vi "Go Home.vi"() -> ()   [LabVIEW 2017]
uses:
  Go Home State type def.ctl
panel:
  out "X-axis distance":dbl
  out "Y-axis distance":dbl
  in  "stop":bool
  out "Motor Status":cluster{"Homing Freq":dbl, "Homing Duty %":dbl} {"Homing Duty %" format="%#_13g"; "Homing Freq" format="%#_13g"}
  in  "Homing Duty %":dbl format="%#_13g"
  in  "Homing Freq":dbl format="%#_13g"
  in  "error in (no error)":errorcluster
  out "error out":errorcluster
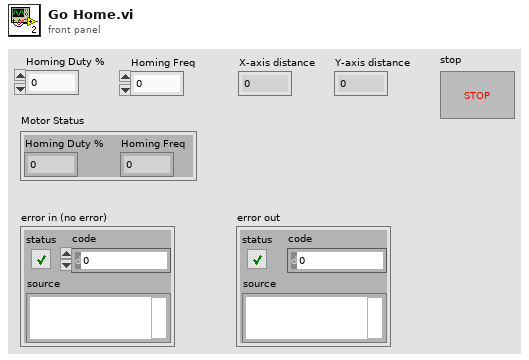
[diagram p1: front panel]
types:
  T1 = typedef "Go Home State type def.ctl" = enum16{"Stop Motor", "Read Input", "Drive Y", "Drive X"}
  T2 = typedef "Encoder Count Direction Enum.ctl" = enum16{"Counting Up", "Counting Down"}
  T3 = cluster{"Y-axis rev count":dbl, "Y-axis distance":dbl, "X-axis rev count":dbl, "X-axis distance":dbl, "Y-axis direction":T2, "X-axis direction":T2, "X-counter val":i32, "Y-counter val":i32}
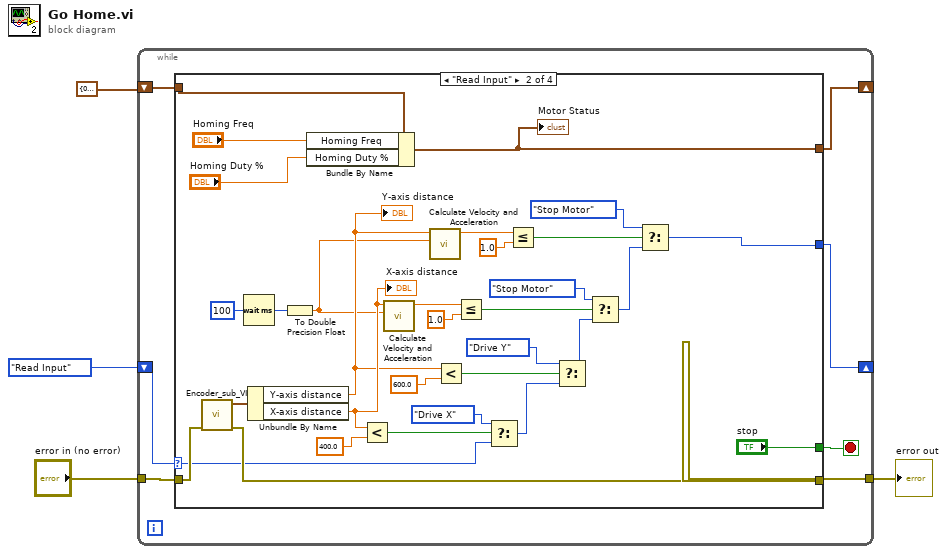
[diagram p0: block diagram]
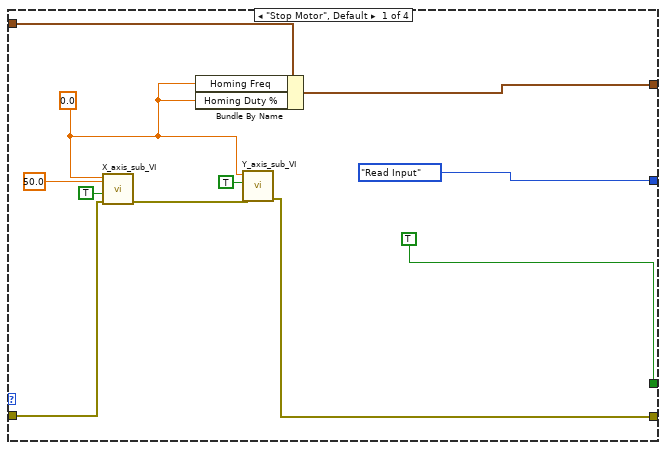
[diagram p2: hidden frame]
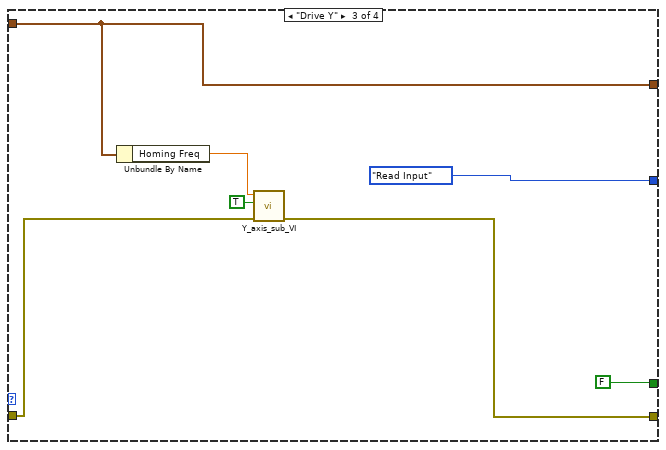
[diagram p3: hidden frame]
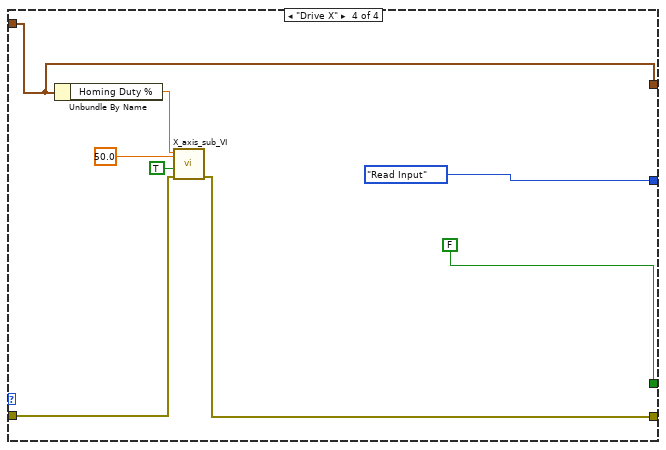
[diagram p4: hidden frame]
diagram:
  n1 = while {
    tunnel: "error in (no error)" -> [w7]
    tunnel: [w6] -> w3
    shift-right: [w8] -> _
    shift-left: Go_Home_State_type_def."Read Input" -> [w11]
    shift-right: [w9] -> _
    shift-left: cluster{"Homing Freq":dbl, "Homing Duty %":dbl} {"Homing Freq"=0.0, "Homing Duty %"=0.0} ("Cluster 2") -> [w10]
    stop <- w5 stop-if-true
    n2 = case shown="\"Read Input\"" w11 {
      selector: w11 -> [_ w38 _ _]
      tunnel: w10 -> [w22 w53 w55 w64]
      tunnel: [w21 w51 w55 w64] -> w9
      tunnel: [Go_Home_State_type_def."Read Input" w25 Go_Home_State_type_def."Read Input" Go_Home_State_type_def."Read Input"] -> w8
      tunnel: w7 -> [w18 w46 w59 w67]
      tunnel: [w19 w45 w58 w66] -> w6
      tunnel: [TRUE "stop" FALSE ("stop") FALSE ("stop")] -> w5
      frame "Stop Motor", Default {
        w17 = 0.0
        n3 = call "X_axis_sub_VI.vi"("error in (no error)"=w18, "FWD/RVS"=TRUE, "Frequency"=50.0, "Duty Cycle %"=w17) -> ("error out"=w20:errorcluster)  [unwired: 7 in]
        n4 = Bundle By Name(cluster=w22, "Homing Freq"=w17, "Homing Duty %"=w17) -> (w21:cluster{"Homing Freq":dbl, "Homing Duty %":dbl})
        n5 = call "Y_axis_sub_VI.vi"("error in (no error)"=w20, "FWD/RVS"=TRUE, "Frequency"=w17) -> ("error out"=w19:errorcluster)  [unwired: 8 in]
      }
      frame "Read Input" {
        n6 = call "Encoder_sub_VI.vi"("error in (no error)"=w46) -> ("error out"=w45:errorcluster, "Encoder Output"=w50:T3)  [unwired: 9 in]
        n7 = Wait (ms)(milliseconds to wait=u32 100) -> (millisecond timer value=w37:u32)
        n8 = Unbundle By Name(w50) -> ("Y-axis distance"=w31:dbl, "X-axis distance"=w36:dbl)
        "Y-axis distance" <- w31
        "X-axis distance" <- w36
        n9 = To Double Precision Float(number=w37) -> (double precision float=w30:dbl)
        n10 = Bundle By Name(cluster=w53, "Homing Freq"="Homing Freq", "Homing Duty %"="Homing Duty %") -> (w51:cluster{"Homing Freq":dbl, "Homing Duty %":dbl})
        "Motor Status" <- w51
        n11 = Less?(x=w36, y=400.0) -> (x < y?=w41:bool)
        n12 = call "Calculate Velocity and Acceleration.vi"("Loop Runtime (s)"=w30, "Displacement (mm)"=w36) -> ("Velocity (mm/s)"=w35:dbl)  [unwired: 8 in, 1 out]
        n13 = call "Calculate Velocity and Acceleration.vi"("Loop Runtime (s)"=w30, "Displacement (mm)"=w31) -> ("Velocity (mm/s)"=w28:dbl)  [unwired: 8 in, 1 out]
        n14 = Less?(x=w31, y=600.0) -> (x < y?=w39:bool)
        n15 = Less Or Equal?(x=w35, y=1.0) -> (x <= y?=w33:bool)
        n16 = Select(t=Go_Home_State_type_def."Drive X", s=w41, f=w38) -> (s? t:f=w48:T1)
        n17 = Less Or Equal?(x=w28, y=1.0) -> (x <= y?=w27:bool)
        n18 = Select(t=Go_Home_State_type_def."Drive Y", s=w39, f=w48) -> (s? t:f=w32:T1)
        n19 = Select(t=Go_Home_State_type_def."Stop Motor", s=w33, f=w32) -> (s? t:f=w26:T1)
        n20 = Select(t=Go_Home_State_type_def."Stop Motor", s=w27, f=w26) -> (s? t:f=w25:T1)
      }
      frame "Drive Y" {
        n21 = Unbundle By Name(w55) -> ("Homing Freq"=w56:dbl)
        n22 = call "Y_axis_sub_VI.vi"("error in (no error)"=w59, "FWD/RVS"=TRUE, "Frequency"=w56) -> ("error out"=w58:errorcluster)  [unwired: 8 in]
      }
      frame "Drive X" {
        n23 = Unbundle By Name(w64) -> ("Homing Duty %"=w65:dbl)
        n24 = call "X_axis_sub_VI.vi"("error in (no error)"=w67, "FWD/RVS"=TRUE, "Frequency"=50.0, "Duty Cycle %"=w65) -> ("error out"=w66:errorcluster)  [unwired: 7 in]
      }
    }
  }
  "error out" <- w3
